vi "Rotate Offset.vi"(10 "Input Vector":dbl[](array[numeric]), 11 "theta":dbl) -> (2 "Output Vector":dbl[](array[numeric]))   [LabVIEW 2011]
uses:
  <vilib>/Analysis/coordinate.llb/2D Cartesian Coordinate Rotation (Scalar).vi
  <vilib>/Analysis/NI_AALPro.lvlib
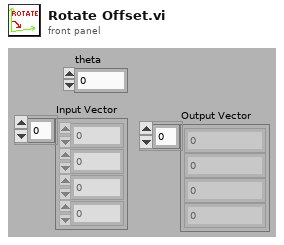
[diagram p1: front panel]
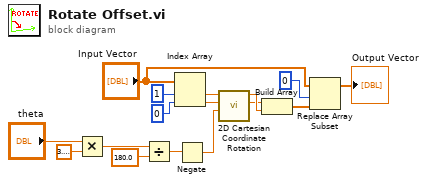
[diagram p0: block diagram]
diagram:
  n1 = Multiply(x="theta", y=3.141592653589793) -> (x*y=w6:dbl)
  n2 = Divide(x=w6, y=180.0) -> (x/y=w2:dbl)
  n3 = Index Array(array="Input Vector", index #1=1 ("index"), index #2=0 ("index")) -> (element #1=w14:dbl, element #2=w13:dbl)
  n4 = Negate(x=w2) -> (-x=w1:dbl)
  n5 = call-poly <vilib>:"2D Cartesian Coordinate Rotation.vi"("theta"=w1, "y"=w13, "x"=w14) -> ("y out"=w10:dbl, "x out"=w11:dbl)  [unwired: 7 out]
  n6 = Build Array(w10, w11) -> (w9:dbl[])
  n7 = Replace Array Subset(array="Input Vector", new element=w9, index=0) -> (→"Output Vector":dbl[])
